vi "Output_ZA.vi"(8 "error in (no error)":errorcluster, 9 "State":string, 10 "Analytics Information":T1, 11 "Zen Analytics in":refnum<class "Zen Analytics.lvclass">) -> (0 "error out":errorcluster, 3 "Zen Analytics out":refnum<class "Zen Analytics.lvclass">)   [LabVIEW 2019, in "Zen Analytics.lvlib" / "Zen Analytics.lvclass"]
uses:
  Zen Analytics.lvclass
  <vilib>/ActorFramework/Actor/Actor.lvclass
  Inspection Statemachine/Inspection Statemachine Messages/Statistics Parameters_SM Msg/Statistics Parameters_SM Msg.lvclass
  Inspection Statemachine/Inspection Statemachine Messages/Acknowledgement_SM Msg/Acknowledgement_SM.lvclass
  Inspection Statemachine/Inspection Statemachine Messages/ErrorMessage_SM Msg/ErrorMessage_SM Msg.lvclass
  C:/Program Files/National Instruments/LabVIEW 2019/vi.lib/ActorFramework/Actor/Actor.lvclass
  <vilib>/ActorFramework/Message Enqueuer/Message Enqueuer.lvclass
  Dependency/GraphReff.ctl
  Dependency/AnalyticsDataToSM.ctl
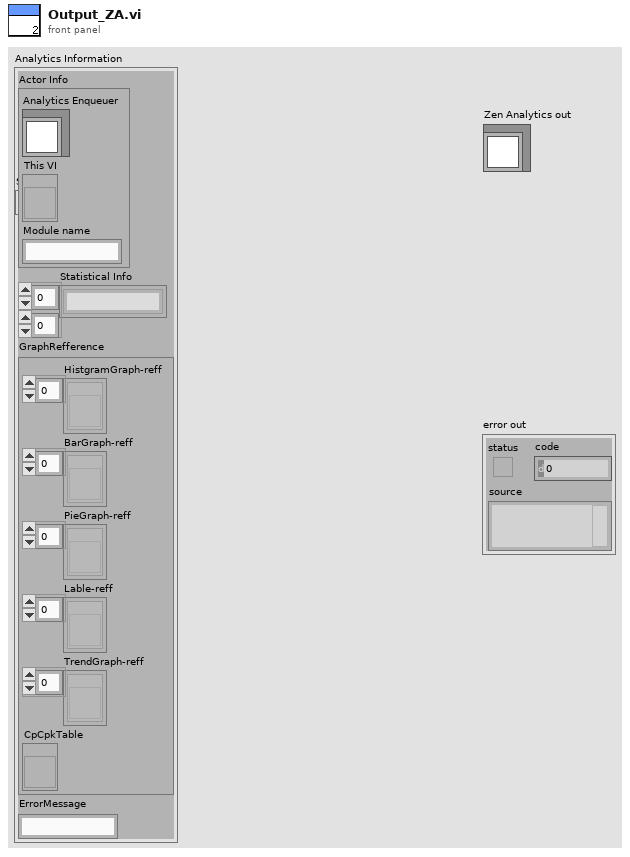
[diagram p1: front panel]
types:
  T1 = typedef "Zen Analytics.lvlib/Zen Analytics.lvclass/AnalyticsDataToSM.ctl" = cluster{"Actor Info":cluster{"Analytics Enqueuer":refnum<class "Message Enqueuer.lvclass">, "This VI":refnum<vi>, "Module name":string}, "Statistical Info":string[][], "Graph Refference's":T2, "ErrorMessage":string}
  T2 = typedef "Zen Analytics.lvlib/Zen Analytics.lvclass/GraphReff.ctl" = cluster{"HistgramGraph-reff":refnum<vi>[], "BarGraph-reff":refnum<vi>[], "PieGraph-reff":refnum<vi>[], "Lable-reff":refnum<vi>[], "TrendGraph-reff":refnum<vi>[], "CpCpkTable":refnum<vi>}
  T3 = cluster{"Analytics Enqueuer":refnum<class "Message Enqueuer.lvclass">, "This VI":refnum<vi>, "Module name":string}
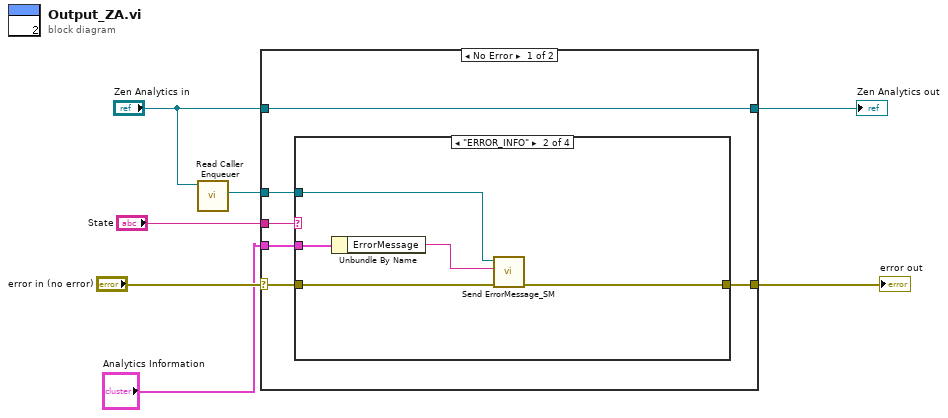
[diagram p0: block diagram]
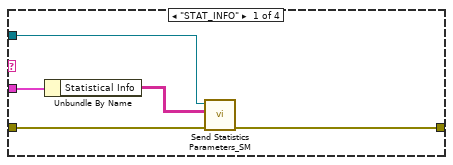
[diagram p2: hidden frame]
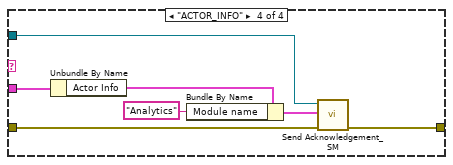
[diagram p4: hidden frame]
diagram:
  n1 = call <vilib>:"Read Caller Enqueuer.vi"("Actor"="Zen Analytics in") -> ("Caller Enqueuer"=w2:refnum<class "Message Enqueuer.lvclass">)  [unwired: 10 in]
  n2 = case shown="No Error" "error in (no error)" {
    selector: "error in (no error)" -> [w9 w33]
    tunnel: [w8 w33] -> w6
    tunnel: [w13 w32] -> w5
    tunnel: "Zen Analytics in" -> [w13 w32]
    tunnel: "State" -> [w12 _]
    tunnel: "Analytics Information" -> [w11 _]
    tunnel: w2 -> [w10 _]
    frame No Error {
      n3 = case shown="\"ERROR_INFO\"" w12 {
        tunnel: w9 -> [w15 w22 w24 w26]
        tunnel: w11 -> [w18 w23 _ w31]
        tunnel: w10 -> [w16 w20 _ w27]
        tunnel: [w14 w21 w24 w25] -> w8
        frame "STAT_INFO" {
          n4 = Unbundle By Name(w18) -> ("Statistical Info"=w17:string[][])
          n5 = call "Send Statistics Parameters_SM.vi"("error in (no error)"=w15, "StatisticalParameters"=w17, "Message Enqueuer"=w16) -> ("error out"=w14:errorcluster)  [unwired: 7 in, 1 out]
        }
        frame "ERROR_INFO" {
          n6 = Unbundle By Name(w23) -> ("ErrorMessage"=w19:string)
          n7 = call "Send ErrorMessage_SM.vi"("error in (no error)"=w22, "Error Message"=w19, "Message Enqueuer"=w20) -> ("error out"=w21:errorcluster)  [unwired: 7 in, 1 out]
        }
        frame Default {
        }
        frame "ACTOR_INFO" {
          n8 = Unbundle By Name(w31) -> ("Actor Info"=w30:T3)
          n9 = Bundle By Name(cluster=w30, "Module name"="Analytics" ("Actor Info.Module name")) -> (w28:T3)
          n10 = call "Send Acknowledgement_SM.vi"("error in (no error)"=w26, "Acknowledgement"=w28, "Message Enqueuer"=w27) -> ("error out"=w25:errorcluster)  [unwired: 7 in, 1 out]
        }
      }
    }
    frame Error {
    }
  }
  "error out" <- w6
  "Zen Analytics out" <- w5
